vi "GetSuffix.vi"(10 "suffix length":i32, 11 "string":string) -> (3 "suffix":string)   [LabVIEW 2015, in "DiffVI.lvclass"]
uses:
  DiffVI.lvclass
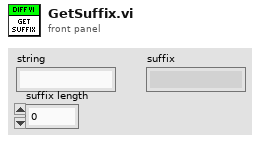
[diagram p1: front panel]
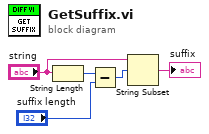
[diagram p0: block diagram]
diagram:
  n1 = String Length(string="string") -> (length=w2:i32)
  n2 = Subtract(x=w2, y="suffix length") -> (x-y=w4:i32)
  n3 = String Subset(string="string", offset (0)=w4) -> (substring=→"suffix":string)  [unwired: 1 in]
